vi "XNET_Frame_InStream_Write.vi"() -> ()   [LabVIEW 2018]
uses:
  <resource>/objmgr/xnet.rc
  <vilib>/xnet/xnet.llb/XNET Frame Type CAN.ctl
  <vilib>/xnet/xnet.llb/XNET Frame CAN.ctl
  <vilib>/xnet/xnet.llb/XNET Create Session (Frame Output Stream).vi
  <vilib>/xnet/xnet.llb/XNET Write (Frame CAN).vi
panel:
  in  "Boolean":bool
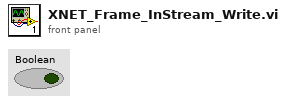
[diagram p1: front panel]
types:
  T1 = typedef "XNET Frame CAN.ctl" = cluster{"timestamp":timestamp, "payload":u8[], "identifier":u32, "type":T2, "extended?":bool, "echo?":bool}
  T2 = typedef "XNET Frame Type CAN.ctl" = u8
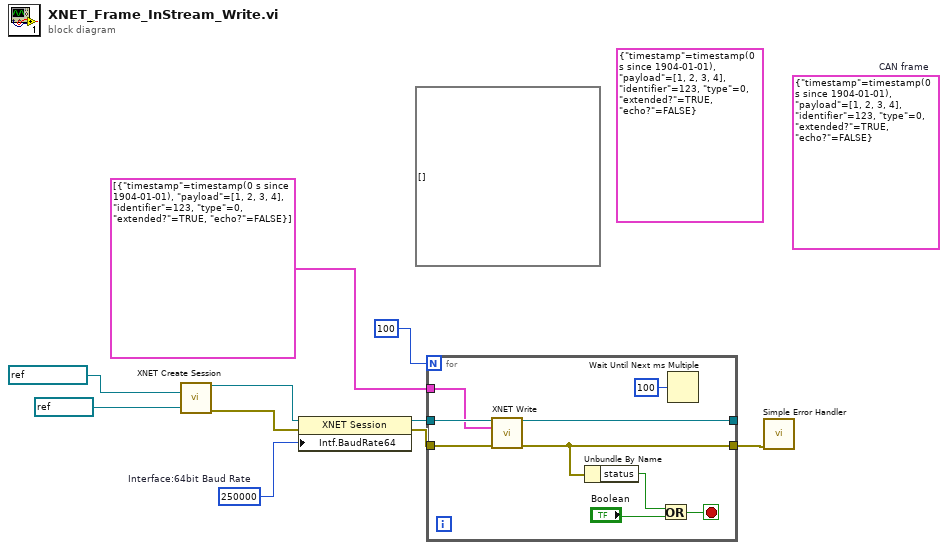
[diagram p0: block diagram]
diagram:
  (unwired) T1 {"timestamp"=timestamp(0 s since 1904-01-01), "payload"=[1, 2, 3, 4], "identifier"=123, "type"=0, "extended?"=TRUE, "echo?"=FALSE}  # CAN frame
  (unwired) T1 {"timestamp"=timestamp(0 s since 1904-01-01), "payload"=[1, 2, 3, 4], "identifier"=123, "type"=0, "extended?"=TRUE, "echo?"=FALSE} ("CAN frame")
  (unwired) void[] [] ("data")
  w8 = u64 250000  # Interface:64bit Baud Rate
  n1 = call-poly <vilib>:"XNET Create Session.vi"("cluster (:memory:)"=refnum<k21> ":memory:", "interface"=refnum<k21> "CAN1") -> ("session out"=w9:refnum<k21>, "error out"=w6:errorcluster)  [unwired: 12 in]
  n2 = property class="XNET Session"(reference=w9, error in=w6, "Intf.BaudRate64"=w8) -> (reference out=w5:refnum<k21>, error out=w4:errorcluster)
  n3 = for {
    N: 100 -> [_]
    tunnel: w5 -> [w13]
    tunnel: w4 -> [w15]
    tunnel: [w12] -> _
    tunnel: [w14] -> w1
    tunnel: T1[] [{"timestamp"=timestamp(0 s since 1904-01-01), "payload"=[1, 2, 3, 4], "identifier"=123, "type"=0, "extended?"=TRUE, "echo?"=FALSE}] ("data") -> [w11]
    stop <- w19 stop-if-true
    n4 = call-poly <vilib>:"XNET Write.vi"("session in"=w13, "data"=w11, "error in (no error)"=w15) -> ("session out"=w12:refnum<k21>, "error out"=w14:errorcluster)  [unwired: 11 in]
    n5 = Unbundle By Name(w14) -> ("status"=w18:bool)
    n6 = Or(x=w18, y="Boolean") -> (x .or. y?=w19:bool)
    n7 = Wait Until Next ms Multiple(millisecond multiple=u32 100) -> ()  [unwired: 1 out]
  }
  n8 = call <vilib>:"Simple Error Handler.vi"("error in (no error)"=w1) -> ()  [unwired: 4 in, 5 out]
